vi "Get one MathCAD design.vi"(8 "error in (no error)":errorcluster) -> (0 "error out":errorcluster, 1 "Number of Pending Requests":i32, 3 "Mathcad Output":T1, 9 "Find-Replace":cluster{"Find":string, "Replace":string}[](array[cluster]), 11 "DesignRequest":T2)   [LabVIEW 2015]
uses:
  AutoCAD cmds.ctl
  AguaClara Library.lvlib
  Word cmd.ctl
  Mathcad Prime cmds.ctl
  Variable cluster.ctl
  Design Request.ctl
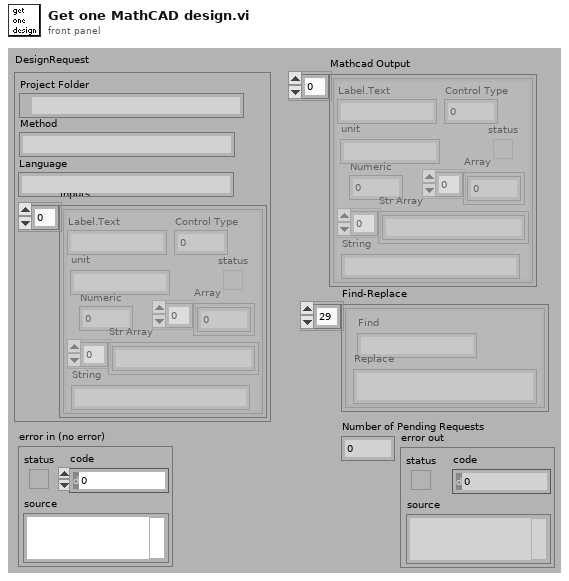
[diagram p1: front panel]
types:
  T1 = typedef "Variable cluster.ctl" = cluster{"Label.Text":string, "Control Type":u32, "Numeric":dbl, "Array":dbl[], "status":bool, "Str Array":string[], "String":string, "unit":string}[]
  T2 = typedef "Design Request.ctl" = cluster{"Project Folder":path, "Method":string, "Inputs":T1, "Language":string}
  T3 = typedef "Mathcad Prime cmds.ctl" = enum16{"Open Mathcad", "Open Worksheet", "Send Inputs", "Read Results", "Quit Mathcad"}
  T4 = typedef "AguaClara Library.lvlib/Word cmd.ctl" = enum16{"Initialize", "Load User Inputs", "Update Fields", "Replace Variables", "Save pdf", "Close Word"}
  T5 = typedef "AguaClara Library.lvlib/AutoCAD cmds.ctl" = enum16{"Open AutoCAD", "New Document", "Send Command", "Send Command Array", "Close Doc", "Quit"}
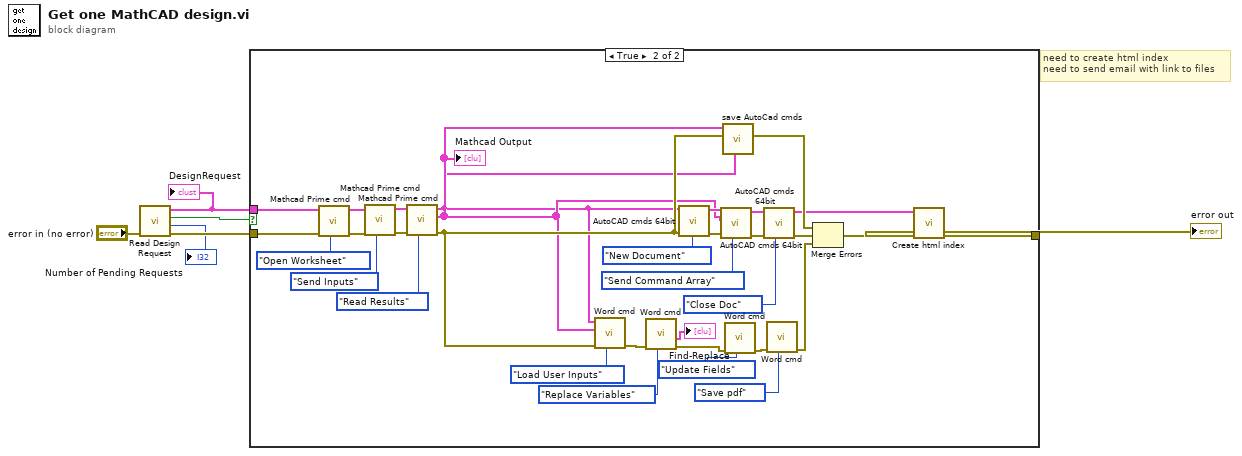
[diagram p0: block diagram]
diagram:
  # "need to create html index\nneed to send email with link to files"
  n1 = call "Read Design Request.vi"("error in"="error in (no error)") -> ("error out"=w4:errorcluster, "Number of Pending Requests"=→"Number of Pending Requests":i32, "Request Pending"=w5:bool, "DesignRequest"=w2:T2)  [unwired: 7 in]
  "DesignRequest" <- w2
  n2 = case shown="True" w5 {
    tunnel: w4 -> [w7 w29]
    tunnel: w2 -> [_ w21]
    tunnel: [w7 w9] -> w1
    frame False {
    }
    frame True {
      n3 = call "Mathcad Prime cmd.vi"("Mathcad Prime cmds"=Mathcad_Prime_cmds."Open Worksheet", "error in (no error)"=w29, "DesignRequest"=w21) -> ("error out"=w27:errorcluster, "DesignRequest out"=w20:T2)  [unwired: 6 in, 1 out]
      n4 = call "Mathcad Prime cmd.vi"("Mathcad Prime cmds"=Mathcad_Prime_cmds."Send Inputs", "error in (no error)"=w27, "DesignRequest"=w20) -> ("error out"=w25:errorcluster, "DesignRequest out"=w19:T2)  [unwired: 6 in, 1 out]
      n5 = call "Mathcad Prime cmd.vi"("Mathcad Prime cmds"=Mathcad_Prime_cmds."Read Results", "error in (no error)"=w25, "DesignRequest"=w19) -> ("error out"=w23:errorcluster, "Mathcad Output"=w15:T1, "DesignRequest out"=w14:T2)  [unwired: 6 in]
      "Mathcad Output" <- w15
      n6 = call "Word cmd.vi"("Word cmd"=Word_cmd."Load User Inputs", "Error In (no error)"=w23, "Mathcad Output"=w15, "DesignRequest"=w14) -> ("error out"=w34:errorcluster)  [unwired: 6 in, 1 out]
      n7 = call "Word cmd.vi"("Word cmd"=Word_cmd."Replace Variables", "Error In (no error)"=w34) -> ("error out"=w13:errorcluster, "Find-Replace"=→"Find-Replace":cluster{"Find":string, "Replace":string}[])  [unwired: 8 in]
      n8 = call "AutoCAD cmds 64bit.vi"("AutoCAD cmd"=AutoCAD_cmds."New Document", "error in (no error)"=w23, "DesignRequest"=w14) -> ("error out"=w37:errorcluster, "DesignRequest out"=w17:T2)  [unwired: 6 in, 1 out]
      n9 = call "AutoCAD cmds 64bit.vi"("AutoCAD cmd"=AutoCAD_cmds."Send Command Array", "error in (no error)"=w37, "Mathcad Output"=w15, "DesignRequest"=w17) -> ("error out"=w40:errorcluster, "DesignRequest out"=w16:T2)  [unwired: 5 in, 1 out]
      n10 = call "save AutoCad cmds.vi"("DesignRequest"=w14, "error in"=w23, "MathCAD results"=w15) -> ("error out"=w22:errorcluster)  [unwired: 8 in]
      n11 = call "Word cmd.vi"("Word cmd"=Word_cmd."Update Fields", "Error In (no error)"=w13) -> ("error out"=w31:errorcluster)  [unwired: 8 in, 1 out]
      n12 = call "AutoCAD cmds 64bit.vi"("AutoCAD cmd"=AutoCAD_cmds."Close Doc", "error in (no error)"=w40, "DesignRequest"=w16) -> ("error out"=w18:errorcluster, "DesignRequest out"=w8:T2)  [unwired: 6 in, 1 out]
      n13 = call "Word cmd.vi"("Word cmd"=Word_cmd."Save pdf", "Error In (no error)"=w31) -> ("error out"=w12:errorcluster)  [unwired: 8 in, 1 out]
      n14 = Merge Errors(w22, w18, w12) -> (w10:errorcluster)
      n15 = call "Create html index.vi"("error in"=w10, "DesignRequest"=w8) -> ("error out"=w9:errorcluster)  [unwired: 9 in]
    }
  }
  "error out" <- w1
